vi "外观.vi"(0 "Data In":T9 caption="数据输入", 2 "Display State In":T2 caption="显示状态输入" {"配置信息"."间隔启动"."启动命令" items=["", "水样测试", "标样核查", "零点核查", "跨度核查", "空白测试", "平行样测试", "加标回收", "空白校准", "标样校准"]; "配置信息"."定点周期"."启动命令 24" items=["", "水样测试", "标样核查", "零点核查", "跨度核查", "空白测试", "平行样测试", "加标回收", "空白校准", "标样校准"]; "配置信息"."定点周期"."启动命令 23" items=["", "水样测试", "标样核查", "零点核查", "跨度核查", "空白测试", "平行样测试", "加标回收", "空白校准", "标样校准"]; "配置信息"."定点周期"."启动命令 22" items=["", "水样测试", "标样核查", "零点核查", "跨度核查", "空白测试", "平行样测试", "加标回收", "空白校准", "标样校准"]; "配置信息"."定点周期"."启动命令 21" items=["", "水样测试", "标样核查", "零点核查", "跨度核查", "空白测试", "平行样测试", "加标回收", "空白校准", "标样校准"]; "配置信息"."定点周期"."启动命令 20" items=["", "水样测试", "标样核查", "零点核查", "跨度核查", "空白测试", "平行样测试", "加标回收", "空白校准", "标样校准"]; "配置信息"."定点周期"."启动命令 19" items=["", "水样测试", "标样核查", "零点核查", "跨度核查", "空白测试", "平行样测试", "加标回收", "空白校准", "标样校准"]; "配置信息"."定点周期"."启动命令 18" items=["", "水样测试", "标样核查", "零点核查", "跨度核查", "空白测试", "平行样测试", "加标回收", "空白校准", "标样校准"]; "配置信息"."定点周期"."启动命令 17" items=["", "水样测试", "标样核查", "零点核查", "跨度核查", "空白测试", "平行样测试", "加标回收", "空白校准", "标样校准"]; "配置信息"."定点周期"."启动命令 16" items=["", "水样测试", "标样核查", "零点核查", "跨度核查", "空白测试", "平行样测试", "加标回收", "空白校准", "标样校准"]; "配置信息"."定点周期"."启动命令 15" items=["", "水样测试", "标样核查", "零点核查", "跨度核查", "空白测试", "平行样测试", "加标回收", "空白校准", "标样校准"]; "配置信息"."定点周期"."启动命令 14" items=["", "水样测试", "标样核查", "零点核查", "跨度核查", "空白测试", "平行样测试", "加标回收", "空白校准", "标样校准"]; "配置信息"."定点周期"."启动命令 13" items=["", "水样测试", "标样核查", "零点核查", "跨度核查", "空白测试", "平行样测试", "加标回收", "空白校准", "标样校准"]; "配置信息"."定点周期"."启动命令 12" items=["", "水样测试", "标样核查", "零点核查", "跨度核查", "空白测试", "平行样测试", "加标回收", "空白校准", "标样校准"]; "配置信息"."定点周期"."启动命令 11" items=["", "水样测试", "标样核查", "零点核查", "跨度核查", "空白测试", "平行样测试", "加标回收", "空白校准", "标样校准"]; "配置信息"."定点周期"."启动命令 10" items=["", "水样测试", "标样核查", "零点核查", "跨度核查", "空白测试", "平行样测试", "加标回收", "空白校准", "标样校准"]; "配置信息"."定点周期"."启动命令 9" items=["", "水样测试", "标样核查", "零点核查", "跨度核查", "空白测试", "平行样测试", "加标回收", "空白校准", "标样校准"]; "配置信息"."定点周期"."启动命令 8" items=["", "水样测试", "标样核查", "零点核查", "跨度核查", "空白测试", "平行样测试", "加标回收", "空白校准", "标样校准"]; "配置信息"."定点周期"."启动命令 7" items=["", "水样测试", "标样核查", "零点核查", "跨度核查", "空白测试", "平行样测试", "加标回收", "空白校准", "标样校准"]; "配置信息"."定点周期"."启动命令 6" items=["", "水样测试", "标样核查", "零点核查", "跨度核查", "空白测试", "平行样测试", "加标回收", "空白校准", "标样校准"]; "配置信息"."定点周期"."启动命令 5" items=["", "水样测试", "标样核查", "零点核查", "跨度核查", "空白测试", "平行样测试", "加标回收", "空白校准", "标样校准"]; "配置信息"."定点周期"."启动命令 4" items=["", "水样测试", "标样核查", "零点核查", "跨度核查", "空白测试", "平行样测试", "加标回收", "空白校准", "标样校准"]; "配置信息"."定点周期"."启动命令 3" items=["", "水样测试", "标样核查", "零点核查", "跨度核查", "空白测试", "平行样测试", "加标回收", "空白校准", "标样校准"]; "配置信息"."定点周期"."启动命令 2" items=["", "水样测试", "标样核查", "零点核查", "跨度核查", "空白测试", "平行样测试", "加标回收", "空白校准", "标样校准"]; "配置信息"."定点周期"."启动命令" items=["", "水样测试", "标样核查", "零点核查", "跨度核查", "空白测试", "平行样测试", "加标回收", "空白校准", "标样校准"]}, 3 "Container State":T8 caption="容器状态") -> (6 "Data Out":T9 caption="数据输出", 7 "Display State Out":T2 caption="显示状态输出" {"配置信息"."间隔启动"."启动命令" items=["", "水样测试", "标样核查", "零点核查", "跨度核查", "空白测试", "平行样测试", "加标回收", "空白校准", "标样校准"]; "配置信息"."定点周期"."启动命令 24" items=["", "水样测试", "标样核查", "零点核查", "跨度核查", "空白测试", "平行样测试", "加标回收", "空白校准", "标样校准"]; "配置信息"."定点周期"."启动命令 23" items=["", "水样测试", "标样核查", "零点核查", "跨度核查", "空白测试", "平行样测试", "加标回收", "空白校准", "标样校准"]; "配置信息"."定点周期"."启动命令 22" items=["", "水样测试", "标样核查", "零点核查", "跨度核查", "空白测试", "平行样测试", "加标回收", "空白校准", "标样校准"]; "配置信息"."定点周期"."启动命令 21" items=["", "水样测试", "标样核查", "零点核查", "跨度核查", "空白测试", "平行样测试", "加标回收", "空白校准", "标样校准"]; "配置信息"."定点周期"."启动命令 20" items=["", "水样测试", "标样核查", "零点核查", "跨度核查", "空白测试", "平行样测试", "加标回收", "空白校准", "标样校准"]; "配置信息"."定点周期"."启动命令 19" items=["", "水样测试", "标样核查", "零点核查", "跨度核查", "空白测试", "平行样测试", "加标回收", "空白校准", "标样校准"]; "配置信息"."定点周期"."启动命令 18" items=["", "水样测试", "标样核查", "零点核查", "跨度核查", "空白测试", "平行样测试", "加标回收", "空白校准", "标样校准"]; "配置信息"."定点周期"."启动命令 17" items=["", "水样测试", "标样核查", "零点核查", "跨度核查", "空白测试", "平行样测试", "加标回收", "空白校准", "标样校准"]; "配置信息"."定点周期"."启动命令 16" items=["", "水样测试", "标样核查", "零点核查", "跨度核查", "空白测试", "平行样测试", "加标回收", "空白校准", "标样校准"]; "配置信息"."定点周期"."启动命令 15" items=["", "水样测试", "标样核查", "零点核查", "跨度核查", "空白测试", "平行样测试", "加标回收", "空白校准", "标样校准"]; "配置信息"."定点周期"."启动命令 14" items=["", "水样测试", "标样核查", "零点核查", "跨度核查", "空白测试", "平行样测试", "加标回收", "空白校准", "标样校准"]; "配置信息"."定点周期"."启动命令 13" items=["", "水样测试", "标样核查", "零点核查", "跨度核查", "空白测试", "平行样测试", "加标回收", "空白校准", "标样校准"]; "配置信息"."定点周期"."启动命令 12" items=["", "水样测试", "标样核查", "零点核查", "跨度核查", "空白测试", "平行样测试", "加标回收", "空白校准", "标样校准"]; "配置信息"."定点周期"."启动命令 11" items=["", "水样测试", "标样核查", "零点核查", "跨度核查", "空白测试", "平行样测试", "加标回收", "空白校准", "标样校准"]; "配置信息"."定点周期"."启动命令 10" items=["", "水样测试", "标样核查", "零点核查", "跨度核查", "空白测试", "平行样测试", "加标回收", "空白校准", "标样校准"]; "配置信息"."定点周期"."启动命令 9" items=["", "水样测试", "标样核查", "零点核查", "跨度核查", "空白测试", "平行样测试", "加标回收", "空白校准", "标样校准"]; "配置信息"."定点周期"."启动命令 8" items=["", "水样测试", "标样核查", "零点核查", "跨度核查", "空白测试", "平行样测试", "加标回收", "空白校准", "标样校准"]; "配置信息"."定点周期"."启动命令 7" items=["", "水样测试", "标样核查", "零点核查", "跨度核查", "空白测试", "平行样测试", "加标回收", "空白校准", "标样校准"]; "配置信息"."定点周期"."启动命令 6" items=["", "水样测试", "标样核查", "零点核查", "跨度核查", "空白测试", "平行样测试", "加标回收", "空白校准", "标样校准"]; "配置信息"."定点周期"."启动命令 5" items=["", "水样测试", "标样核查", "零点核查", "跨度核查", "空白测试", "平行样测试", "加标回收", "空白校准", "标样校准"]; "配置信息"."定点周期"."启动命令 4" items=["", "水样测试", "标样核查", "零点核查", "跨度核查", "空白测试", "平行样测试", "加标回收", "空白校准", "标样校准"]; "配置信息"."定点周期"."启动命令 3" items=["", "水样测试", "标样核查", "零点核查", "跨度核查", "空白测试", "平行样测试", "加标回收", "空白校准", "标样校准"]; "配置信息"."定点周期"."启动命令 2" items=["", "水样测试", "标样核查", "零点核查", "跨度核查", "空白测试", "平行样测试", "加标回收", "空白校准", "标样校准"]; "配置信息"."定点周期"."启动命令" items=["", "水样测试", "标样核查", "零点核查", "跨度核查", "空白测试", "平行样测试", "加标回收", "空白校准", "标样校准"]}, 8 "Action":T1 caption="动作")   [LabVIEW 2016, in "定时设置.xctl"]
uses:
  <vilib>/_xctls/Container State.ctl
  <vilib>/_xctls/Action.ctl
  <vilib>/Utility/miscctls.llb/LVPositionTypeDef.ctl
  <vilib>/_xctls/XControlSupport.lvlib
  <vilib>/ptbypt/NI_PtbyPt.lvlib
panel:
  in  "周期设置":bool
  # "分钟"
  # "次"
  # "分钟"
  # "次"
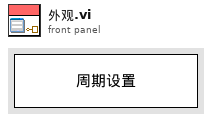
[diagram p1: front panel]
types:
  T1 = typedef "XControlSupport.lvlib/Action.ctl" = cluster{"Data Changed?":bool, "State Changed?":bool, "Action Name":string}
  T2 = typedef "定时设置.xctl/状态.ctl" = cluster{"配置信息":cluster{"周期模式":T3, "定点周期":T4, "间隔启动":T6, "测量参数":T7}, "仪器运行状态":bool, "启动次数":i32, "最近一次启动时间":timestamp, "最近一次结束时间":timestamp, "间隔计时":dbl, "重写配置文件":bool, "测量参数名称":string[]}
  T3 = typedef "定时设置.xctl/周期模式设置.ctl" = enum16{"不启用", "定点模式", "间隔模式"}
  T4 = typedef "定时设置.xctl/定点周期设置.ctl" = cluster{"启动命令":T5, "启动命令 2":T5, "启动命令 3":T5, "启动命令 4":T5, "启动命令 5":T5, "启动命令 6":T5, "启动命令 7":T5, "启动命令 8":T5, "启动命令 9":T5, "启动命令 10":T5, "启动命令 11":T5, "启动命令 12":T5, "启动命令 13":T5, "启动命令 14":T5, "启动命令 15":T5, "启动命令 16":T5, "启动命令 17":T5, "启动命令 18":T5, "启动命令 19":T5, "启动命令 20":T5, "启动命令 21":T5, "启动命令 22":T5, "启动命令 23":T5, "启动命令 24":T5}
  T5 = typedef "定时设置.xctl/启动命令选择.ctl" = u16
  T6 = typedef "定时设置.xctl/间隔启动设置.ctl" = cluster{"启动命令":T5, "启动间隔":dbl, "启动次数":i32}
  T7 = typedef "定时设置.xctl/测量参数.ctl" = u16
  T8 = typedef "XControlSupport.lvlib/Container State.ctl" = cluster{"Indicator?":bool, "Run Mode?":bool, " Refnum":refnum<vi>}
  T9 = typedef "定时设置.xctl/数据.ctl" = cluster{"启动":bool, "控制命令":T10, "测量参数":T7}
  T10 = typedef "定时设置.xctl/国标控制命令.ctl" = enum16{"启动测量", "标样核查", "零点核查", "跨度核查", "空白测试", "平行样测试", "加标回收", "空白校准", "标样校准", "初始化（清洗）", "停止测试", "仪器重启", "校时", "模式设置", "测量间隔设置"}
  T11 = typedef "LVPositionTypeDef.ctl" = cluster{"Left":i32, "Top":i32}
  T12 = cluster{"周期模式":T3, "定点周期":T4, "间隔设置":cluster{"启动命令":T5, "启动间隔":dbl, "启动次数":i32}, "测量参数":T7}
  T13 = cluster{"周期模式":T3, "定点周期":T4, "间隔启动":T6, "测量参数":T7}
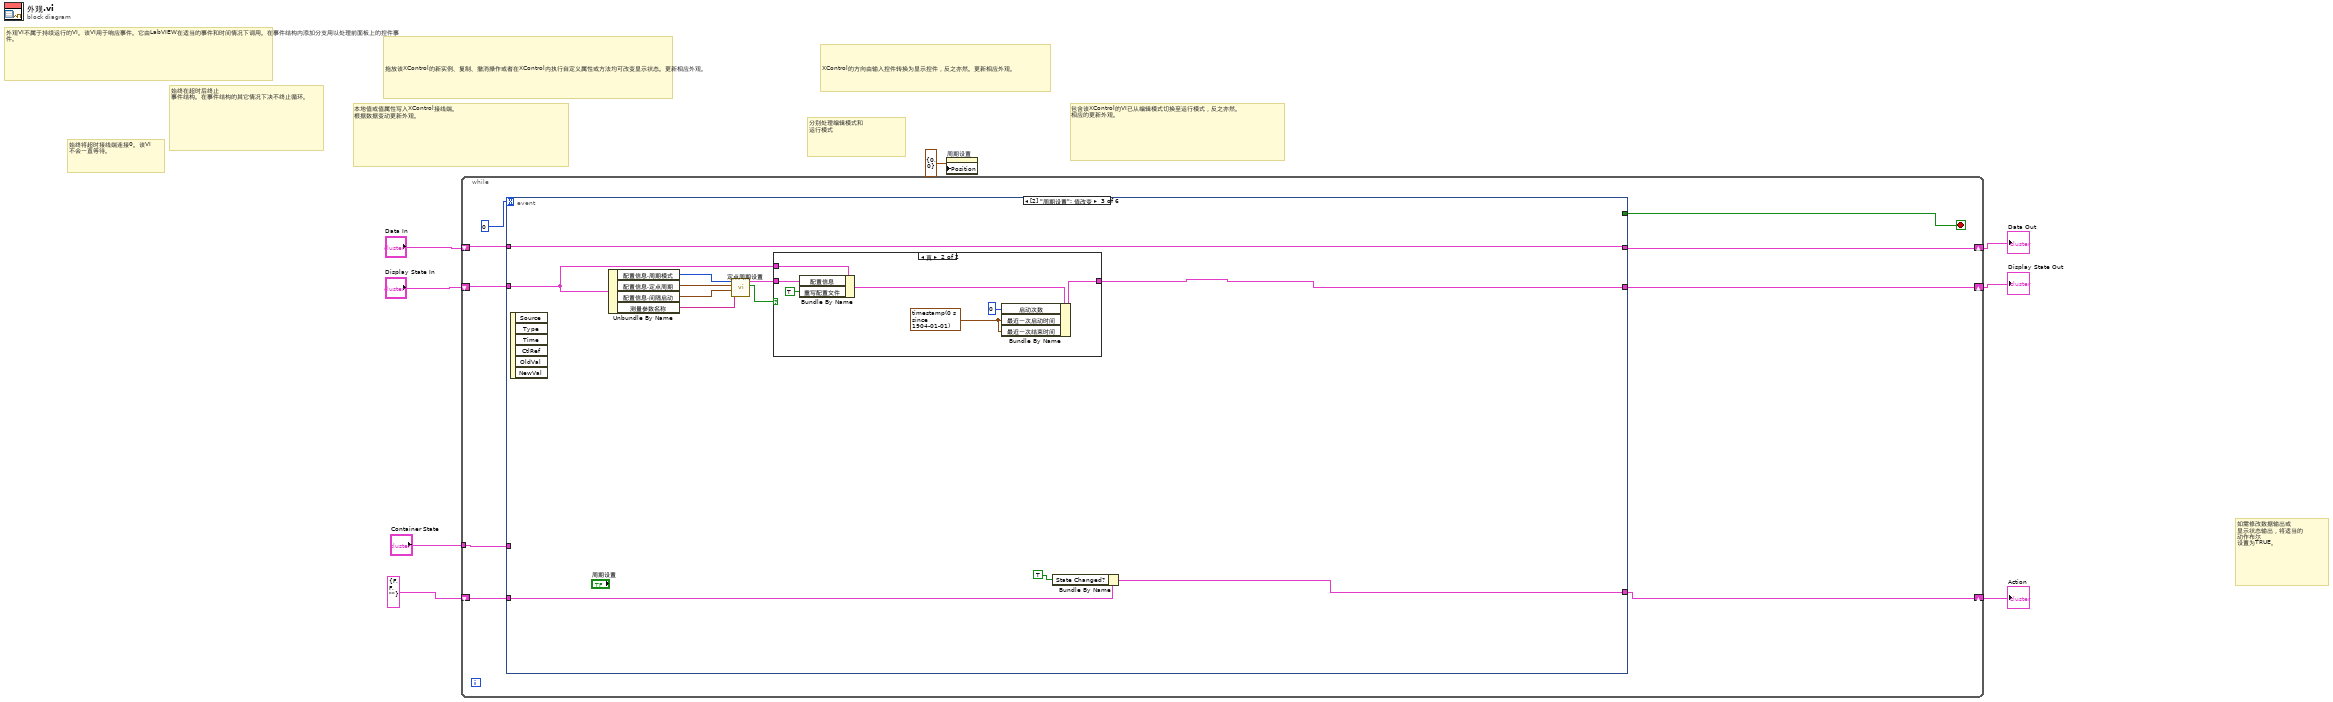
[diagram p0: block diagram]
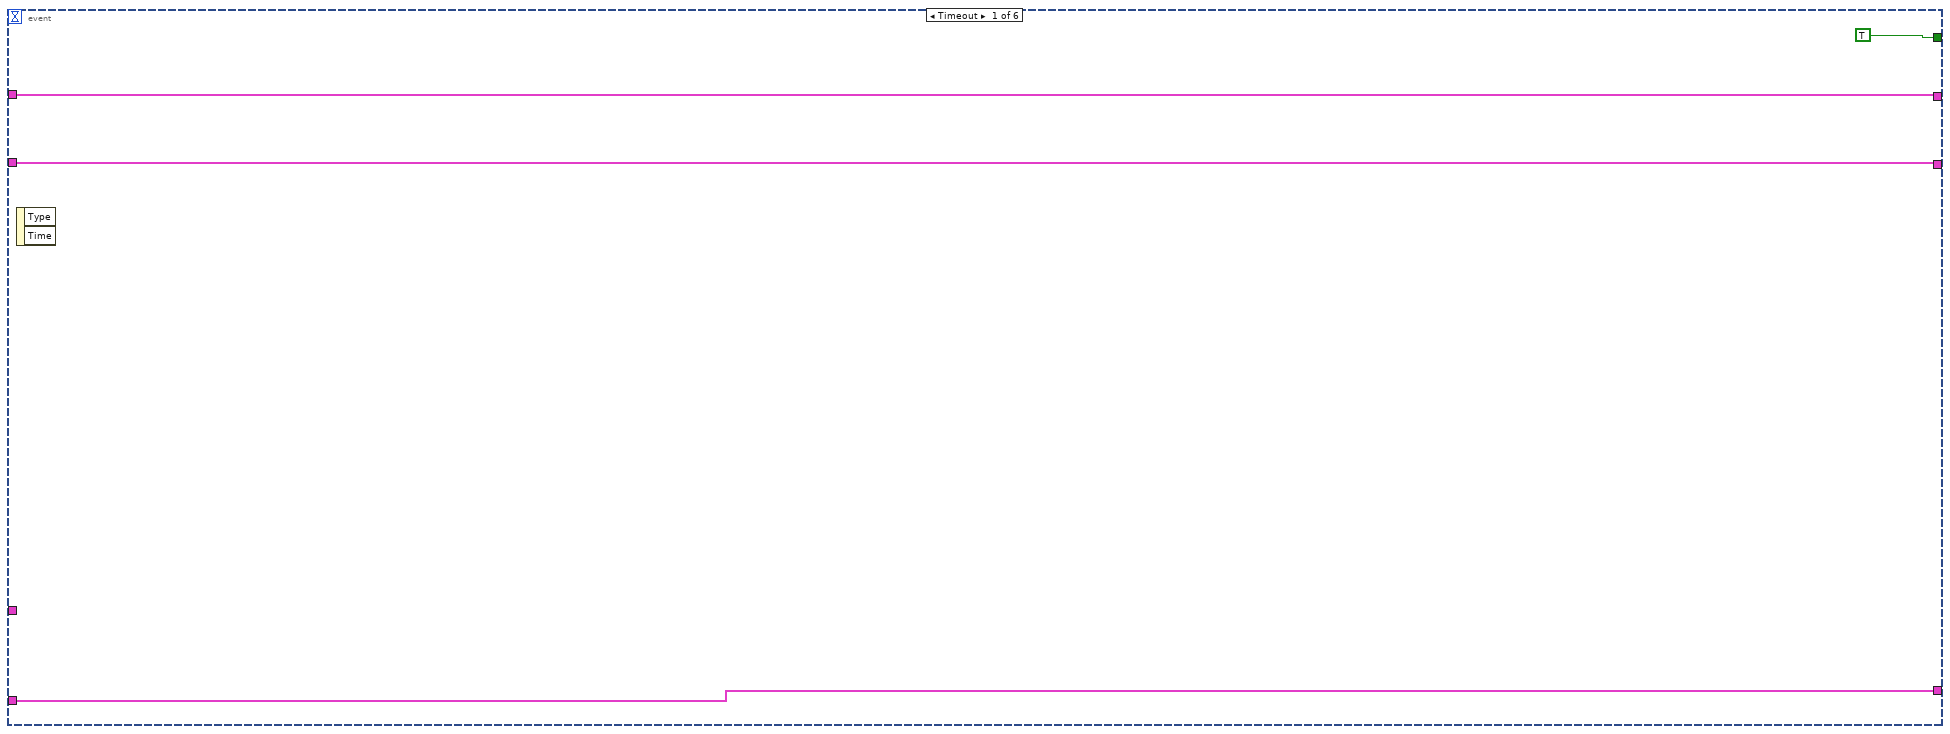
[diagram p2: hidden frame]
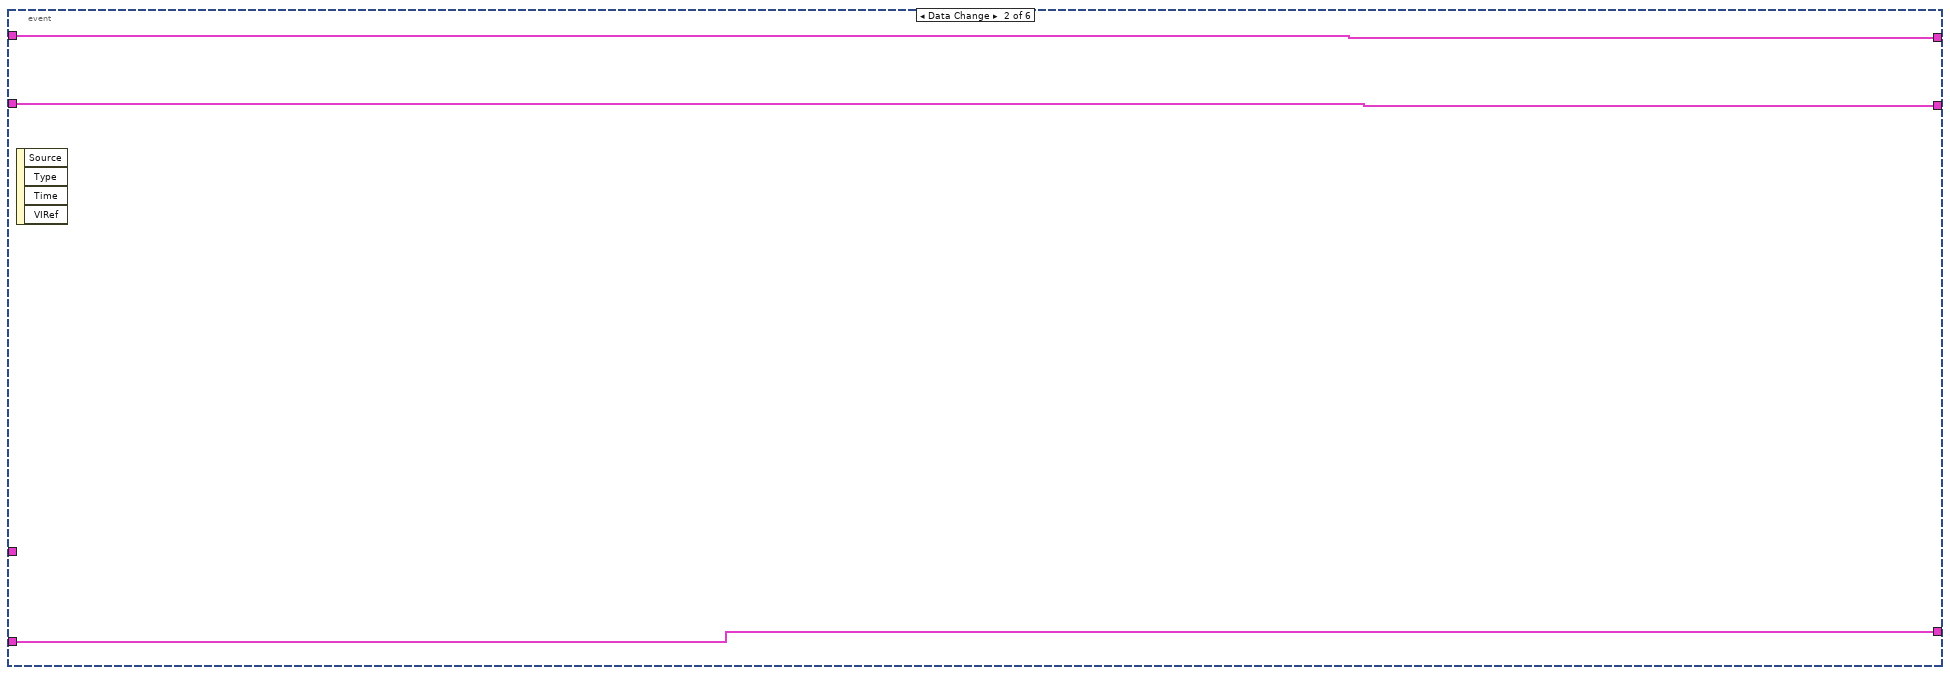
[diagram p3: hidden frame]
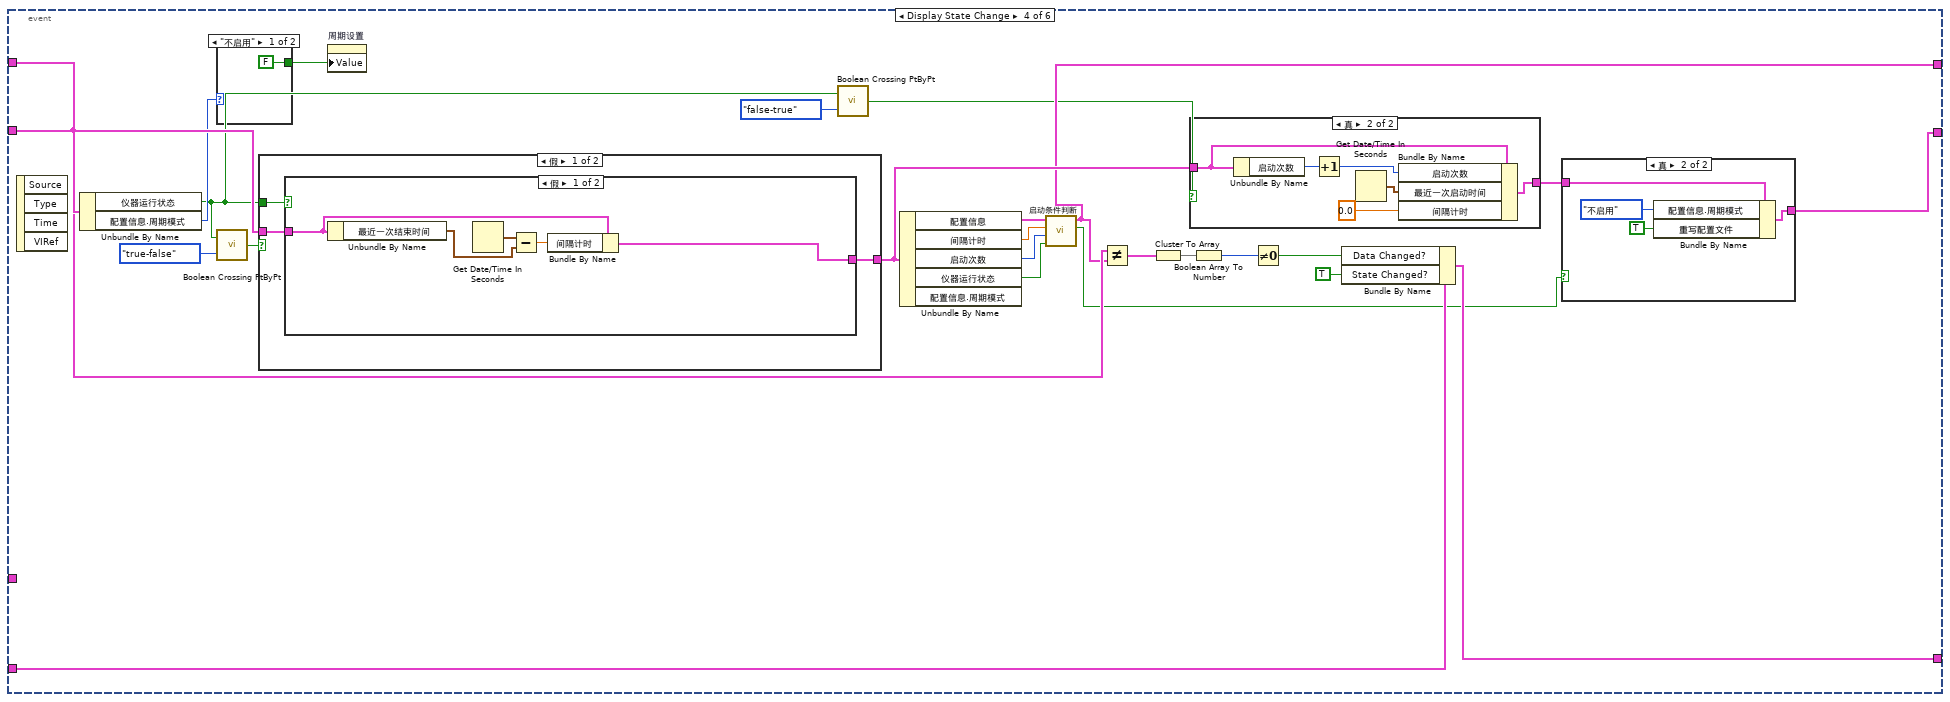
[diagram p5: hidden frame]
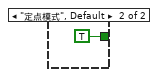
[diagram p7: hidden frame]
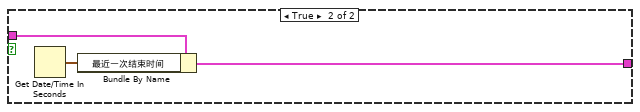
[diagram p9: hidden frame]
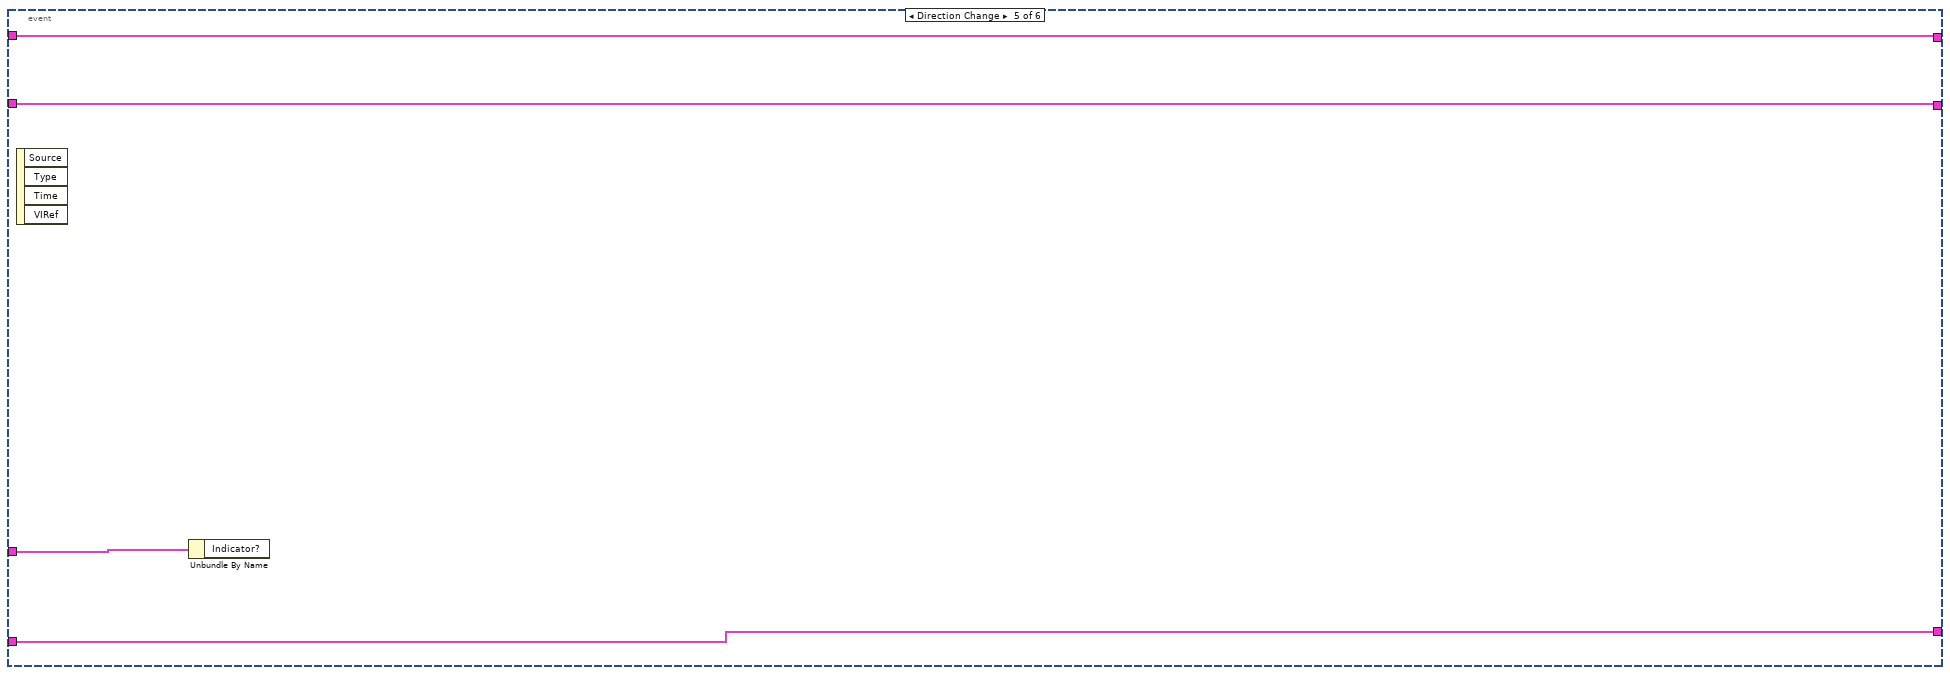
[diagram p11: hidden frame]
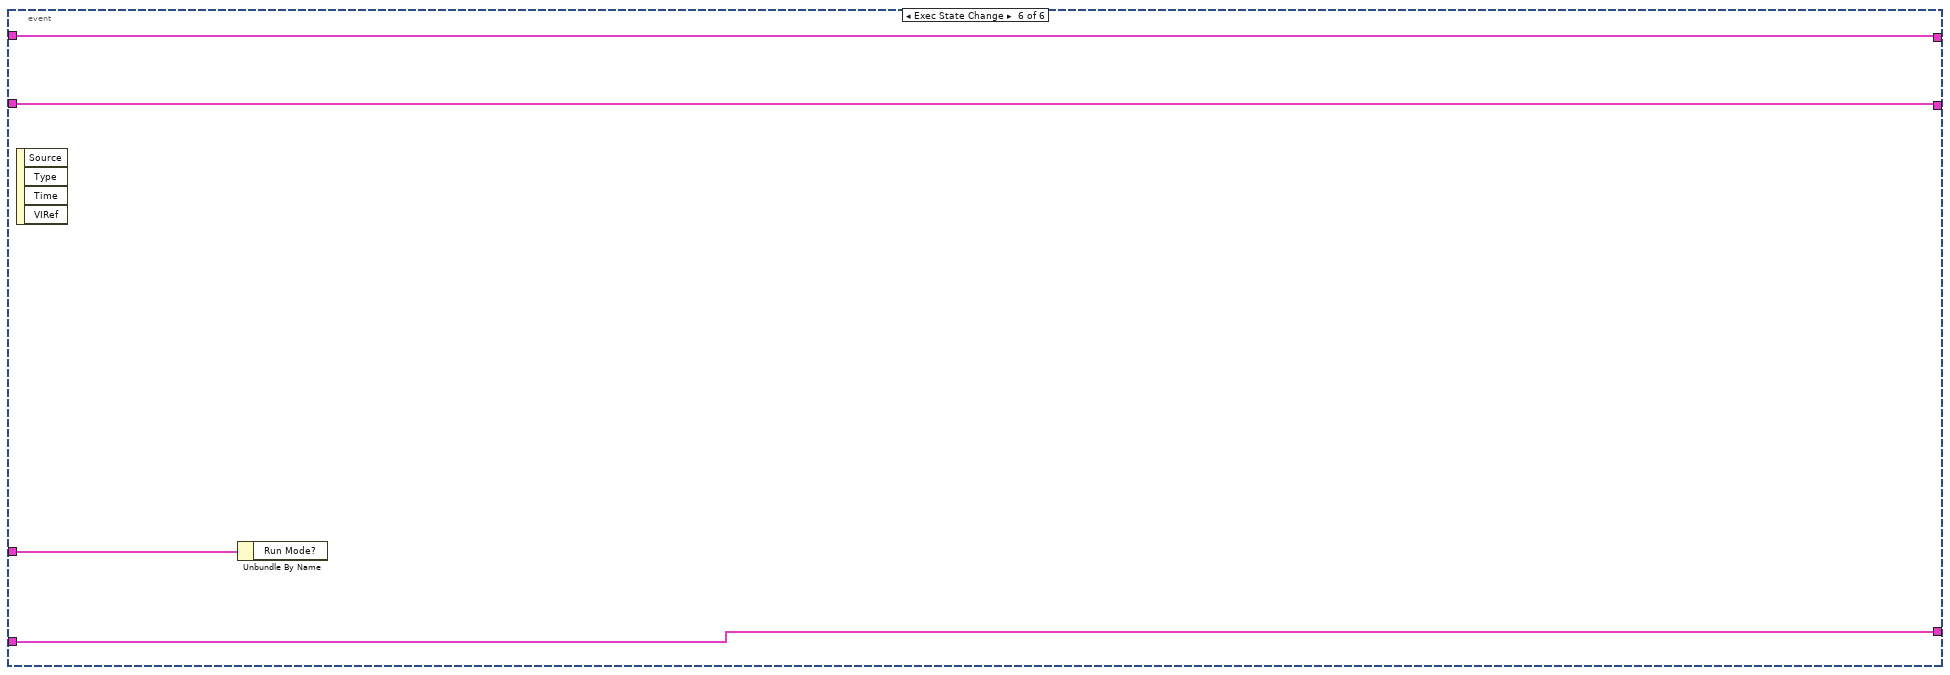
[diagram p12: hidden frame]
diagram:
  # "分别处理编辑模式和\n运行模式"
  # "包含该XControl的VI已从编辑模式切换至运行模式，反之亦然。\n相应的更新外观。"
  # "XControl的方向由输入控件转换为显示控件，反之亦然。更新相应外观。"
  # "始终将超时接线端连接0。该VI\n不会一直等待。"
  # "拖放该XControl的新实例、复制、撤消操作或者在XControl内执行自定义属性或方法均可改变显示状态。更新相应外观。"
  # "本地值或值属性写入XControl接线端。\n根据数据变动更新外观。"
  # "始终在超时后终止\n事件结构。在事件结构的其它情况下决不终止循环。"
  # "外观VI不属于持续运行的VI。该VI用于响应事件。它由LabVIEW在适当的事件和时间情况下调用。在事件结构内添加分支用以处理前面板上的控件事件。"
  # "如需修改数据输出或\n显示状态输出，将适当的\n动作布尔\n设置为TRUE。"
  n1 = while {
    shift-right: [w16] -> w5
    shift-left: "Display State In" -> [w17]
    tunnel: "Container State" -> [w13]
    shift-right: [w11] -> w8
    shift-left: "Data In" -> [w12]
    shift-right: [w9] -> w3
    shift-left: T1 {"Data Changed?"=FALSE, "State Changed?"=FALSE, "Action Name"=""} ("Action") -> [w10]
    stop <- w15 stop-if-true
    n2 = event shown="[2] \"周期设置\": 值改变" {
      selector: _ -> [_ _ _ _ _ _]
      dyn-events: _ -> [_ _ _ _ _ _]
      timeout: 0 -> [_ _ _ _ _ _]
      tunnel: w17 -> [w19 w23 w33 w64 w98 w102]
      tunnel: [w19 w23 w26 w48 w98 w102] -> w16
      tunnel: [TRUE _ _ _ _ _] -> w15
      tunnel: w13 -> [_ _ _ _ w99 w103]
      tunnel: w12 -> [w18 w24 w34 w56 w97 w101]
      tunnel: [w18 w24 w34 w55 w97 w101] -> w11
      tunnel: [w20 w22 w31 w67 w96 w100] -> w9
      tunnel: w10 -> [w20 w22 w32 w68 w96 w100]
      event Timeout {
        n3 = event-data() -> ()  [unwired: 1 in, 2 out]
      }
      event Data Change {
        n4 = event-data() -> ()  [unwired: 1 in, 4 out]
      }
      event "周期设置": Value Change {
        n5 = event-data() -> ()  [unwired: 1 in, 6 out]
        n6 = Unbundle By Name(w33) -> ("配置信息.周期模式"=w28:T3, "配置信息.定点周期"=w35:T4, "配置信息.间隔启动"=w36:T6, "测量参数名称"=w25:string[])
        n7 = call "定点周期设置.vi"("测量参数字符串[]"=w25, "间隔启动"=w36, "定点周期"=w35, "周期模式"=w28) -> ("保存输出"=w27:bool, "周期设置输出"=w29:T12)  [unwired: 6 in]
        n8 = case shown="真" w27 {
          tunnel: w33 -> [w37 w44]
          tunnel: [w37 w41] -> w26
          tunnel: w29 -> [_ w42]
          frame False {
          }
          frame True {
            w40 = timestamp(0 s since 1904-01-01) ("最近一次启动时间")
            n9 = Bundle By Name(cluster=w44, "配置信息"=w42, "重写配置文件"=TRUE) -> (w43:T2)
            n10 = Bundle By Name(cluster=w43, "启动次数"=0, "最近一次启动时间"=w40, "最近一次结束时间"=w40) -> (w41:T2)
          }
        }
        n11 = Bundle By Name(cluster=w32, "State Changed?"=TRUE) -> (w31:T1)
      }
      event Display State Change {
        n12 = event-data() -> ()  [unwired: 1 in, 4 out]
        n13 = Unbundle By Name(w64) -> ("仪器运行状态"=w46:bool, "配置信息.周期模式"=w58:T3)
        n14 = case shown="\"不启用\"" w58 {
          tunnel: [FALSE TRUE] -> w57
          frame "不启用" {
          }
          frame "定点模式", Default {
          }
        }
        n15 = call <vilib>:"Boolean Crossing PtByPt.vi"("direction"=enum16{"either", "false-true", "true-false"}."true-false", "input"=w46) -> ("crossing"=w65:bool)  [unwired: 1 in]
        n16 = case shown="假" w65 {
          tunnel: w64 -> [w79 w88]
          tunnel: [w78 w87] -> w63
          tunnel: w46 -> [w77 _]
          frame False {
            n17 = case shown="假" w77 {
              tunnel: w79 -> [w83 w85]
              tunnel: [w81 w85] -> w78
              frame False {
                n18 = Unbundle By Name(w83) -> ("最近一次结束时间"=w80:timestamp)
                n19 = Get Date/Time In Seconds() -> (seconds since 1Jan1904=w84:timestamp)
                n20 = Subtract(x=w84, y=w80) -> (x-y=w82:dbl)
                n21 = Bundle By Name(cluster=w83, "间隔计时"=w82) -> (w81:T2)
              }
              frame True {
              }
            }
          }
          frame True {
            n22 = Get Date/Time In Seconds() -> (seconds since 1Jan1904=w86:timestamp)
            n23 = Bundle By Name(cluster=w88, "最近一次结束时间"=w86) -> (w87:T2)
          }
        }
        n24 = property on="周期设置" class="Bool (严格)"("Value"=w57) -> ()  [unwired: 2 in, 2 out]
        n25 = call <vilib>:"Boolean Crossing PtByPt.vi"("direction"=enum16{"either", "false-true", "true-false"}."false-true", "input"=w46) -> ("crossing"=w45:bool)  [unwired: 1 in]
        n26 = Unbundle By Name(w63) -> ("配置信息"=w62:T13, "间隔计时"=w61:dbl, "启动次数"=w60:i32, "仪器运行状态"=w59:bool)  [unwired: 1 out]
        n27 = call "启动条件判断.vi"("仪器状态"=w59, "启动次数"=w60, "间隔计时"=w61, "周期设置输出"=w62) -> ("重新配置"=w49:bool, "Data"=w55:T9)  [unwired: 6 in]
        n28 = Not Equal?(x=w56, y=w55) -> (x != y?=w54:cluster{"启动":bool, "控制命令":bool, "测量参数":bool})
        n29 = Cluster To Array(cluster=w54) -> (array=w53:bool[])
        n30 = case shown="真" w45 {
          tunnel: w63 -> [w89 w93]
          tunnel: [w89 w95] -> w50
          frame False {
          }
          frame True {
            n31 = Unbundle By Name(w93) -> ("启动次数"=w92:i32)
            n32 = Increment(x=w92) -> (x+1=w91:i32)
            n33 = Get Date/Time In Seconds() -> (seconds since 1Jan1904=w94:timestamp)
            n34 = Bundle By Name(cluster=w93, "启动次数"=w91, "最近一次启动时间"=w94, "间隔计时"=0.0) -> (w95:T2)
          }
        }
        n35 = Boolean Array To Number(Boolean array=w53) -> (number=w52:u32)
        n36 = Not Equal To 0?(x=w52) -> (x != 0?=w51:bool)
        n37 = Bundle By Name(cluster=w68, "Data Changed?"=w51, "State Changed?"=TRUE) -> (w67:T1)
        n38 = case shown="真" w49 {
          tunnel: w50 -> [w70 w74]
          tunnel: [w70 w72] -> w48
          frame False {
          }
          frame True {
            n39 = Bundle By Name(cluster=w74, "配置信息.周期模式"=周期模式设置."不启用", "重写配置文件"=TRUE) -> (w72:T2)
          }
        }
      }
      event Direction Change {
        n40 = event-data() -> ()  [unwired: 1 in, 4 out]
        n41 = Unbundle By Name(w99) -> ()  [unwired: 1 out]
      }
      event Exec State Change {
        n42 = event-data() -> ()  [unwired: 1 in, 4 out]
        n43 = Unbundle By Name(w103) -> ()  [unwired: 1 out]
      }
    }
  }
  "Display State Out" <- w5
  "Data Out" <- w8
  "Action" <- w3
  n44 = property on="周期设置" class="Bool (严格)"("Position"=T11 {"Left"=0, "Top"=0} ("位置")) -> ()  [unwired: 2 in, 2 out]
